vi "Register Events.vi"(8 "error in (no error)":errorcluster, 11 "PluginGUI in":refnum<class "PluginGUI.lvclass">) -> (0 "error out":errorcluster, 3 "PluginGUI out":refnum<class "PluginGUI.lvclass">)   [LabVIEW 2020, in "VolatusGUI.lvlib" / "PluginGUI.lvclass"]
uses:
  PluginGUI.lvclass
  PluginGUI.lvclass/PluginGUI.ctl
  Control/Control.lvclass
  Control Event.ctl
  VolatusGUI.lvlib
  <vilib>/Utility/miscctls.llb/LVMapReplaceAction.ctl
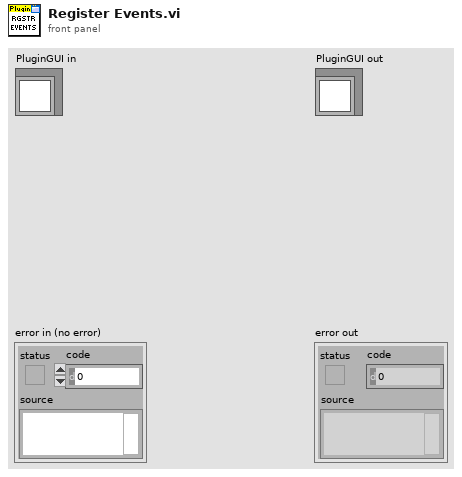
[diagram p1: front panel]
types:
  T1 = typedef "VolatusGUI.lvlib/Control Event.ctl" = enum16{"Value Change", "Shortcut Menu", "Mouse Down"}
  T2 = typedef "LVMapReplaceAction.ctl" = enum32{"Modify Entry only if found", "Add or Modify Entry", "Delete Entry"}
  T3 = typedef "VolatusGUI.lvlib/Event Registration.ctl" = cluster{"CtlRef":refnum<vi>, "Event":T1}
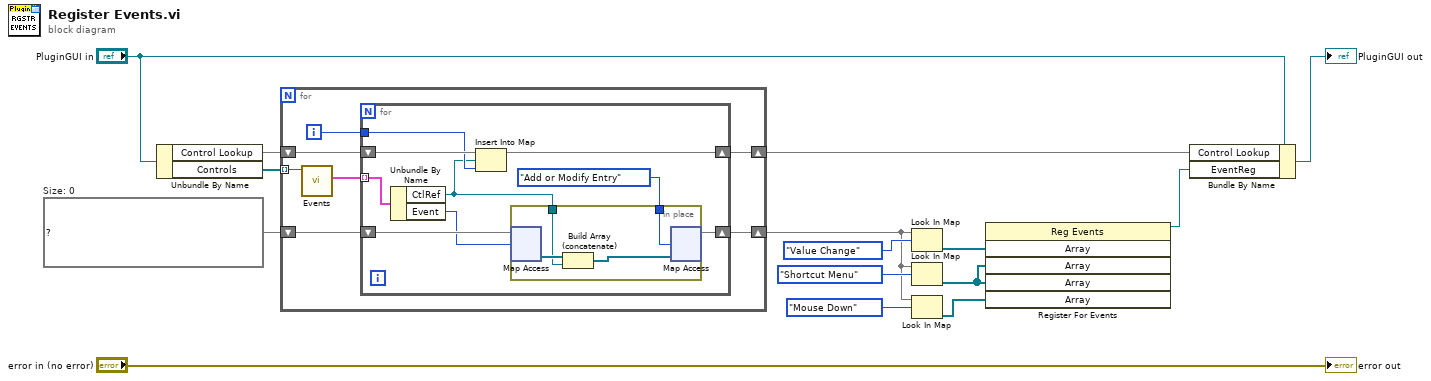
[diagram p0: block diagram]
diagram:
  w12 = map{T1, refnum<vi>[]} {}  # Size: 0
  n1 = Unbundle By Name("PluginGUI in") -> ("Control Lookup"=w13:map{refnum<vi>, i32}, "Controls"=w14:refnum<class "Control.lvclass">[])
  n2 = for {
    tunnel: w14 -> [w22] mode=indexing
    shift-right: [w17] -> w6
    shift-left: w13 -> [w21]
    shift-right: [w16] -> w3
    shift-left: w12 -> [w19]
    i -> [w18]
    n3 = call "Events.vi"("Control in"=w22) -> ("Events"=w20:T3[])  [unwired: 10 in]
    n4 = for {
      shift-right: [w28] -> w17
      shift-left: w21 -> [w30]
      tunnel: w20 -> [w31] mode=indexing
      shift-right: [w23] -> w16
      shift-left: w19 -> [w27]
      tunnel: w18 -> [w29]
      n5 = Unbundle By Name(w31) -> ("CtlRef"=w25:refnum<vi>, "Event"=w26:T1)
      n6 = Insert Into Map(map in=w30, key=w25, value=w29) -> (map out=w28:map{refnum<vi>, i32})  [unwired: 2 out]
      n7 = in-place {
        in-place-border: w25 -> [w34]
        in-place-border: LVMapReplaceAction."Add or Modify Entry" ("action") -> [w32]
        n8 = in-place-map #1(w27, w26) -> (w35:refnum<vi>[])  [unwired: 1 in, 1 out]
        n9 = Build Array (concatenate)(w35, w34) -> (w33:refnum<vi>[])
        n10 = in-place-map #1(w33, w32) -> (w23:map{T1, refnum<vi>[]})  [unwired: 2 out]
      }
    }
  }
  n11 = Look In Map(map=w3, key=Control_Event."Value Change") -> (value=w9:refnum<vi>[])  [unwired: 1 in, 1 out]
  n12 = Look In Map(map=w3, key=Control_Event."Shortcut Menu") -> (value=w8:refnum<vi>[])  [unwired: 1 in, 1 out]
  n13 = Look In Map(map=w3, key=Control_Event."Mouse Down") -> (value=w1:refnum<vi>[])  [unwired: 1 in, 1 out]
  n14 = register-events(w9, w8, w8, w1) -> (reference out=w5:refnum<event-registration>)  [unwired: 2 in, 1 out]
  n15 = Bundle By Name(cluster="PluginGUI in", "Control Lookup"=w6, "EventReg"=w5) -> (→"PluginGUI out":refnum<class "PluginGUI.lvclass">)
  "error out" <- "error in (no error)"
